vi "Main.vi"() -> ()   [LabVIEW 2012]
uses:
  MeasureDialogButton.ctl
  SourceDialogButton.ctl
  TriggerDialogButton.ctl
  DUTDisplayData.ctl
  DUTDialogButton.ctl
  LogDialogButton.ctl
  driver/Public/Controls/SMU.ctl
  DisplayDataGlobalAction.ctl
  UIActionQueueElement.ctl
  UIAction.ctl
  SetupGlobalAction.ctl
  HardwareActionQueueElement.ctl
  HardwareAction.ctl
  HardwareAbortGlobalAction.ctl
  LogActionQueueElement.ctl
  LogAction.ctl
  DisplayDataChartDialogGlobalAction.ctl
  driver/Keithley-2602.lvlib
  libs/LV-Utilities/LV-Utilities.lvlib
panel:
  in  "CREATE PLOT":bool
  in  "Hardware START":bool
  out "Hardware Running?":bool
  in  "LOG START":bool
  out "Log Running?":bool
  out "Digital IO Port":bool[](array[boolean])
  out "Setup File":path
  in  "RESET":bool
  in  "SAVE":bool
  in  "OPEN":bool
  in  "SHOW LOG DIALOG":T1
  in  "SHOW DUT DIALOG":T2
  in  "SHOW SOURCE DIALOG":T3
  in  "SHOW TRIGGER DIALOG":T4
  in  "SHOW MEASURE DIALOG":T5
  out "System SMU B DUT Display Data":T6[](array[typedef]) {"Resistance (Ohm)" format="%_4p"; "Current (A)" format="%_4p"; "Voltage (V)" format="%_4p"}
  out "System SMU A DUT Display Data":T6[](array[typedef]) {"Resistance (Ohm)" format="%_4p"; "Current (A)" format="%_4p"; "Voltage (V)" format="%_4p"}
  out "Log File":path
  in  "DONE":bool
  # "RUN"
  # "LOG"
  # "DIGITAL IO"
  # "1"
  # "2"
  # "3"
  # "4"
  # "5"
  # "6"
  # "7"
  # "8"
  # "9"
  # "10"
  # "11"
  # "12"
  # "13"
  # "14"
  # "SETUP"
  # "SMU B"
  # "SMU A"
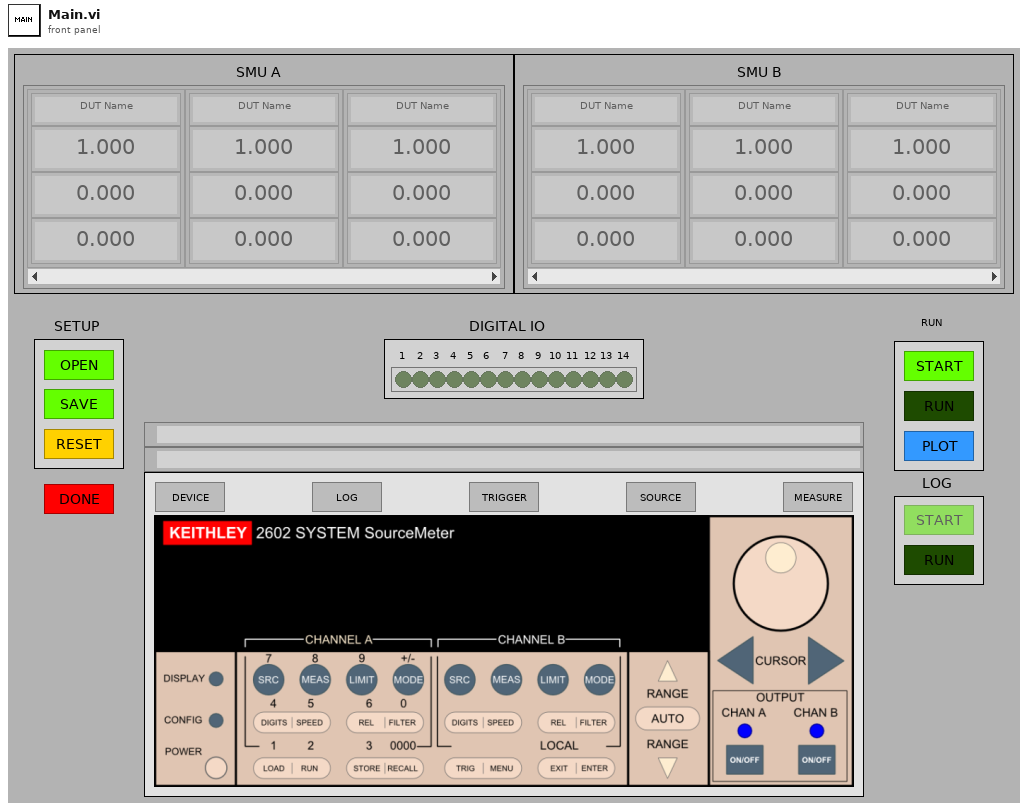
[diagram p1: front panel]
types:
  T1 = typedef "LogDialogButton.ctl" = bool
  T2 = typedef "DUTDialogButton.ctl" = bool
  T3 = typedef "SourceDialogButton.ctl" = bool
  T4 = typedef "TriggerDialogButton.ctl" = bool
  T5 = typedef "MeasureDialogButton.ctl" = bool
  T6 = typedef "DUTDisplayData.ctl" = cluster{"Name":string, "Voltage (V)":dbl, "Current (A)":dbl, "Resistance (Ohm)":dbl}
  T7 = typedef "ExecutableConfiguration.ctl" = cluster{"GPIB ID":u8, "GPIB Board":u8, "Default Data Folder":path, "Default Setup Folder":path}
  T8 = typedef "DataStructures.ctl" = cluster{"Display Data":refnum<notifier>, "Log Data":refnum<queue>}
  T9 = typedef "ActionQueues.ctl" = cluster{"UI Action":refnum<queue>, "Hardware Action":refnum<queue>, "Log Action":refnum<queue>}
  T10 = typedef "DisplayDataGlobalAction.ctl" = enum16{"Get", "Set"}
  T11 = typedef "Keithley-2602.lvlib/SMU.ctl" = enum16{"A", "B"}
  T12 = typedef "SetupGlobalAction.ctl" = enum16{"Get", "Set", "Reset"}
  T13 = enum8{"Enabled", "Disabled", "Disabled and Grayed Out"}
  T14 = typedef "UIActionQueueElement.ctl" = cluster{"Action":T15, "Data":variant}
  T15 = typedef "UIAction.ctl" = enum16{"Initialize", "Configure Trigger", "Configure Measure", "Configure Source", "Configure DUT", "Configure Log", "Configure Open", "Configure Save", "Configure Reset", "Hardware Start", "Hardware Started", "Hardware Stop", "Hardware Stopped", "Log Arm", "Log Start", "Log Started", "Log Stop", "Log Stopped", "Create Chart", "Error", "Shutdown"}
  T16 = typedef "HardwareActionQueueElement.ctl" = cluster{"Action":T17, "Data":variant}
  T17 = typedef "HardwareAction.ctl" = enum16{"Initialize", "Start", "Run", "Stop", "Error", "Shutdown"}
  T18 = typedef "HardwareAbortGlobalAction.ctl" = enum16{"Set", "Get"}
  T19 = typedef "LogActionQueueElement.ctl" = cluster{"Action":T20, "Data":variant}
  T20 = typedef "LogAction.ctl" = enum16{"Initialize", "Start", "Arm", "Create", "Write", "Close", "Rearm", "Stop", "Error", "Shutdown"}
  T21 = typedef "DisplayDataChartDialogGlobalAction.ctl" = enum16{"Create", "Close All"}
  T22 = typedef "HardwareDisplayData.ctl" = cluster{"DUT Names":string[][], "SMU":dbl[][], "Port":bool[]}
  T23 = typedef "Setup.ctl" = cluster{"DUT":T24, "Log":T26, "Trigger":T34, "Sources":T40[], "Measures":T42[]}
  T24 = typedef "DUTConfiguration.ctl" = cluster{"Count":u32, "Wirings":T25[], "Names":string[][]}
  T25 = typedef "Keithley-2602.lvlib/SMUSense.ctl" = enum16{"Local (2-wire)", "Remote (4-wire)", "Calibration"}
  T26 = typedef "LogConfiguration.ctl" = cluster{"Start":T27, "Rollover":T30, "Stop":T32}
  T27 = typedef "LogStartConfiguration.ctl" = cluster{"Trigger Type":T28, "Timer (sec)":dbl, "Digital IO Line":u8, "Digital IO Edge":T29}
  T28 = typedef "LogStartTriggerType.ctl" = enum16{"Immediate", "User", "Timer", "Digital IO"}
  T29 = typedef "LogDigitalIOTriggerEdge.ctl" = enum16{"Rising", "Falling"}
  T30 = typedef "LogRolloverConfiguration.ctl" = cluster{"Trigger Type":T31, "Timer (sec)":dbl, "File Size (MB)":u32, "Digital IO Line":u8, "Digital IO Edge":T29}
  T31 = typedef "LogRolloverTriggerType.ctl" = enum16{"None", "Timer", "File Size", "Digital IO"}
  T32 = typedef "LogStopConfiguration.ctl" = cluster{"Trigger Type":T33, "Timer (sec)":dbl, "File Size (MB)":u32, "Digital IO Line":u8, "Digital IO Edge":T29}
  T33 = typedef "LogStopTriggerType.ctl" = enum16{"None", "User", "Timer", "File Size", "Digital IO"}
  T34 = typedef "TriggerConfiguration.ctl" = cluster{"Input":T35, "Output":T38}
  T35 = typedef "TriggerInputConfiguration.ctl" = cluster{"Type":T36, "Timeout (ms)":u32, "Delay (ms)":u32, "Digital IO Line (1-14)":u8, "Digital IO Mode":T37}
  T36 = typedef "TriggerInputType.ctl" = enum16{"None", "Digital IO", "Bus"}
  T37 = typedef "Keithley-2602.lvlib/TriggerMode.ctl" = enum16{"Falling", "Rising", "Either", "Synchronous"}
  T38 = typedef "TriggerOutputConfiguration.ctl" = cluster{"Type":T39, "Delay (ms)":u32, "Digital IO Line (1-14)":u8, "Digital IO Mode":T37, "Digital IO Pulse Width (sec)":dbl}
  T39 = typedef "TriggerOutputType.ctl" = enum16{"None", "Digital IO", "Bus"}
  T40 = typedef "SourceConfiguration.ctl" = cluster{"Enabled?":bool, "Function":T41, "Level (V or A)":dbl, "Autorange Enabled?":bool, "High Limit (V or A)":dbl, "Low Limit (V or A)":dbl}
  T41 = typedef "SourceFunction.ctl" = enum16{"Voltage", "Current"}
  T42 = typedef "MeasureConfiguration.ctl" = cluster{"Enabled?":bool, "Count":u8, "Interval (sec)":dbl, "Voltage Auto Range Enabled?":bool, "Voltage High Limit (V or A)":dbl, "Voltage Low Limit (V or A)":dbl, "Current Auto Range Enabled?":bool, "Current High Limit (V or A)":dbl, "Current Low Limit (V or A)":dbl}
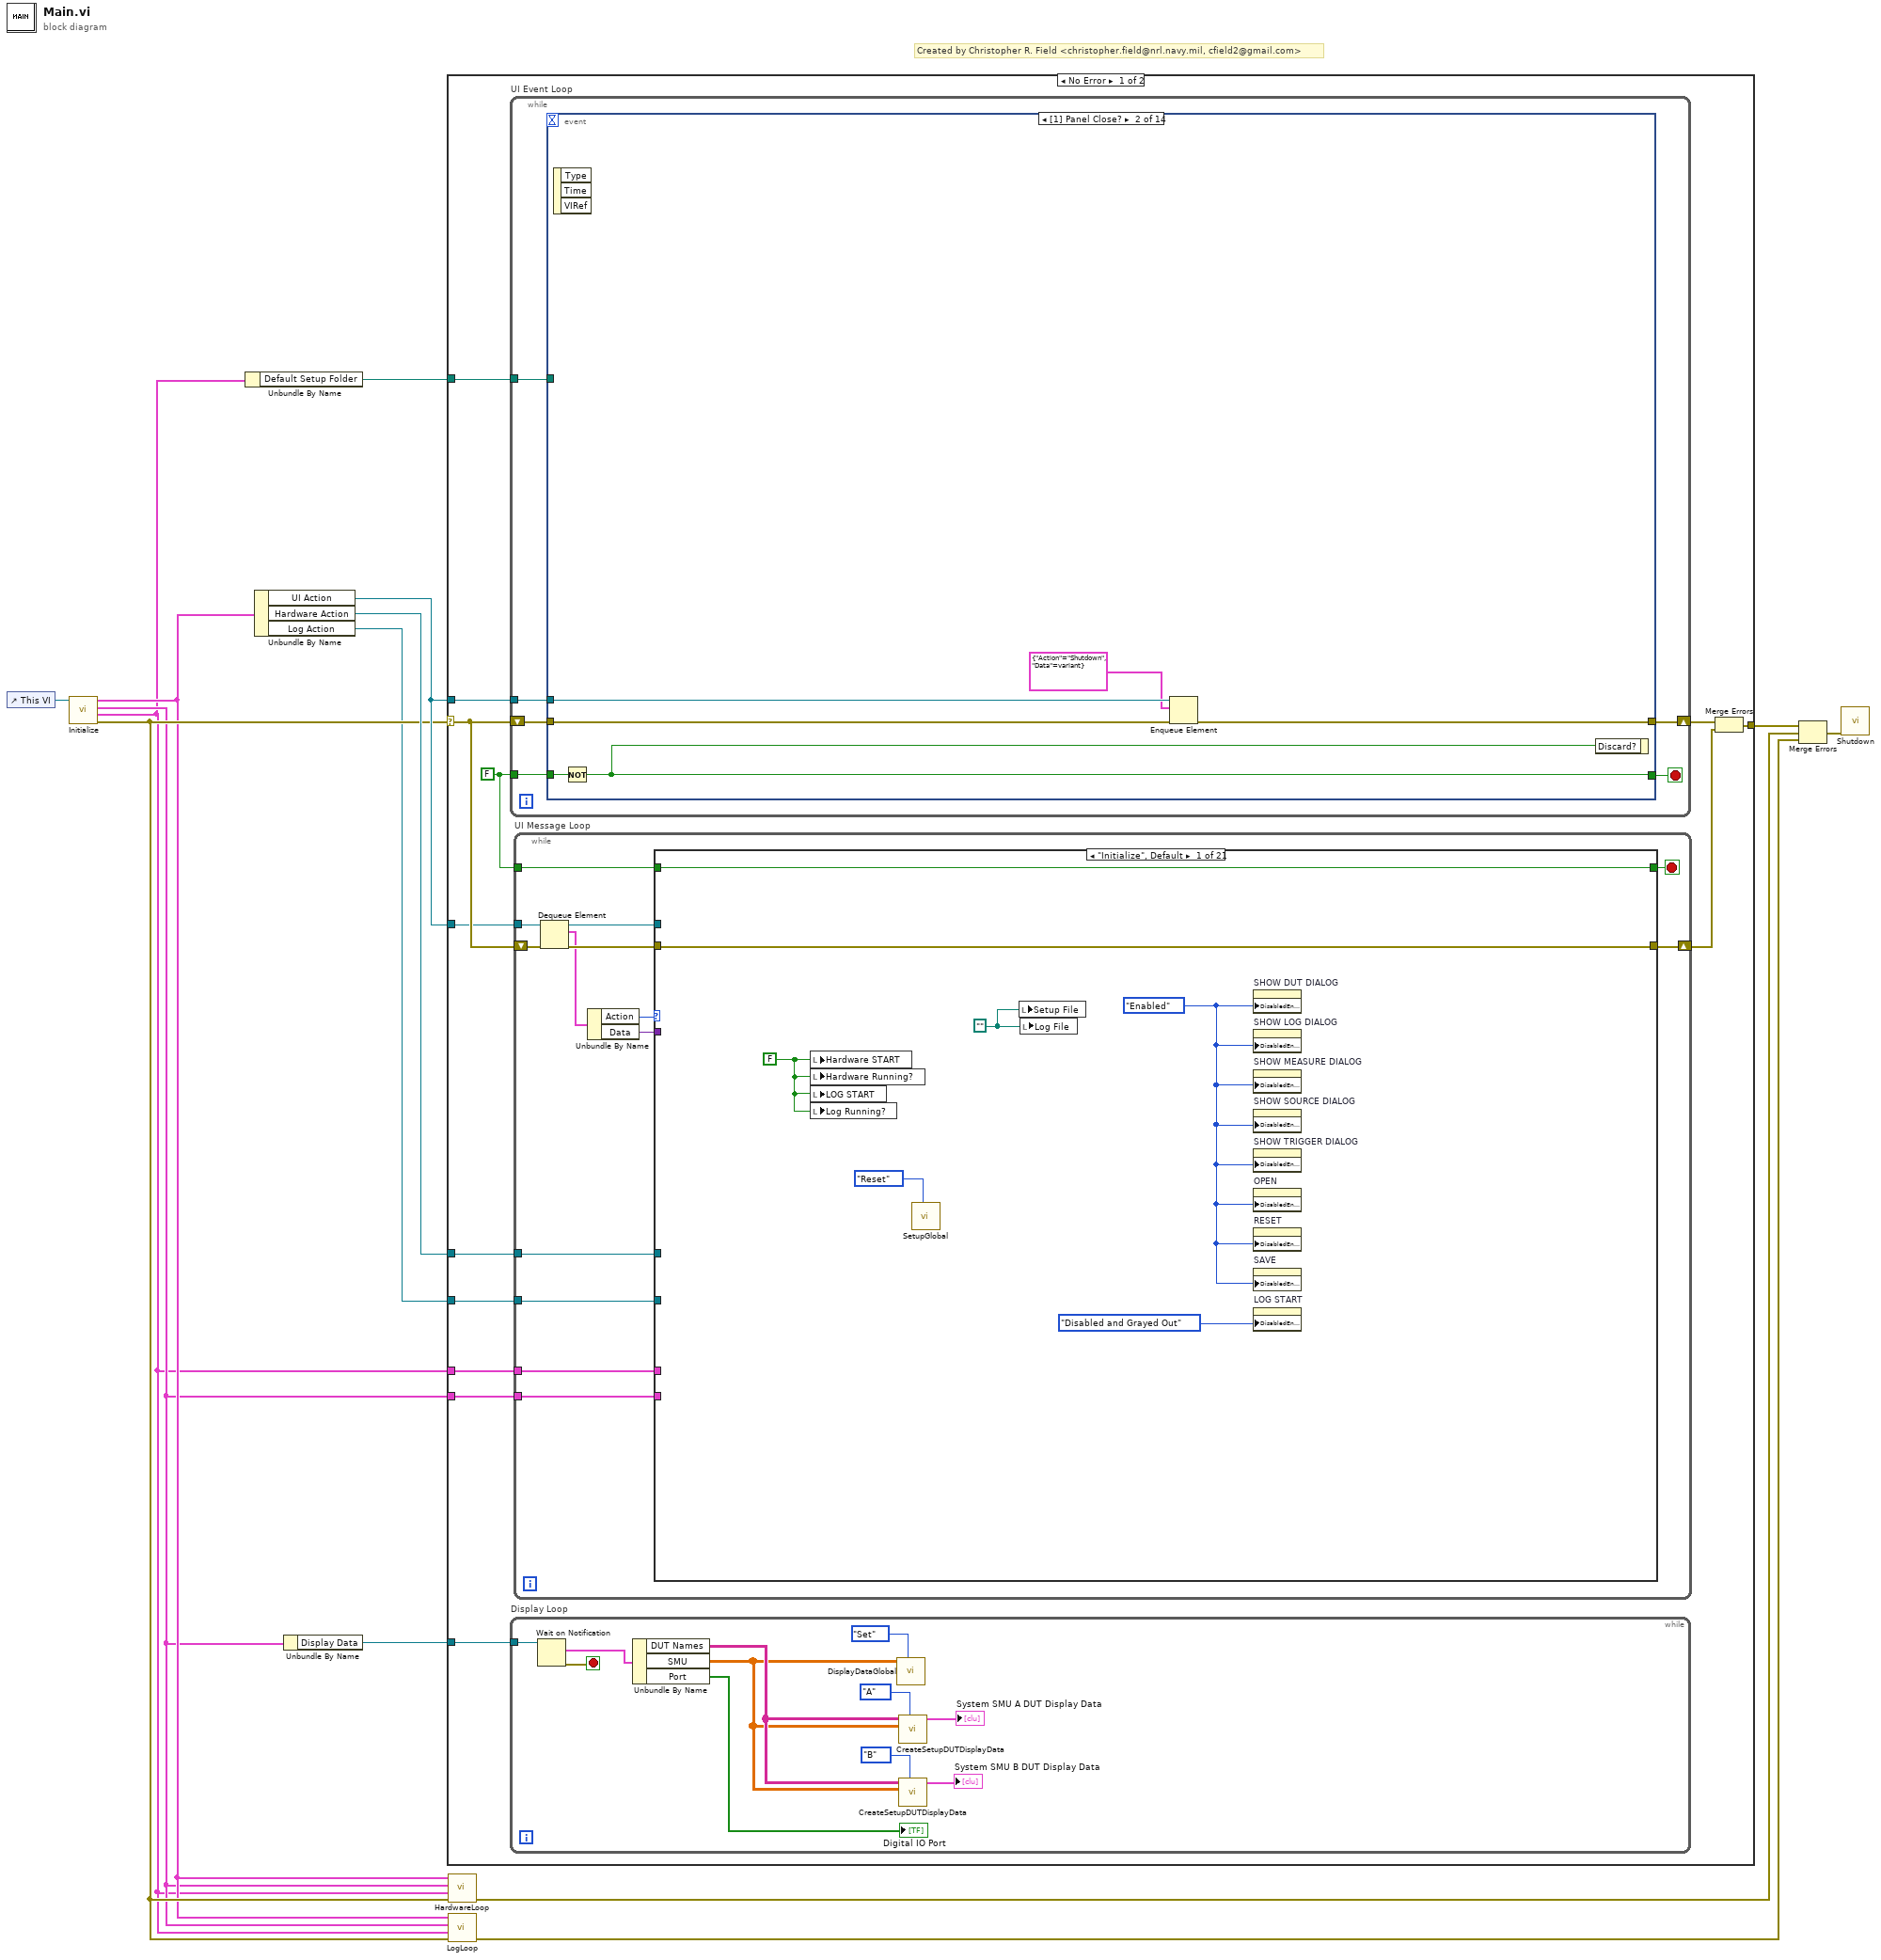
[diagram p0: block diagram]
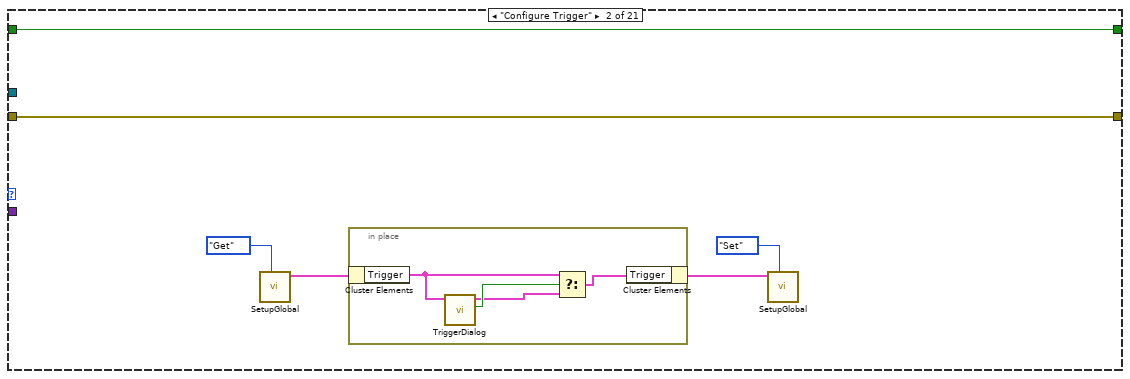
[diagram p2: hidden frame]
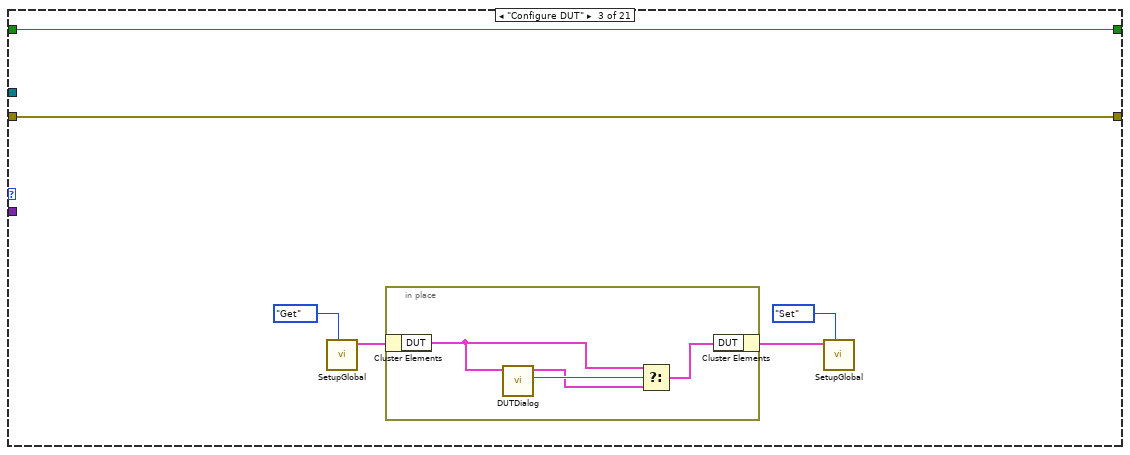
[diagram p3: hidden frame]
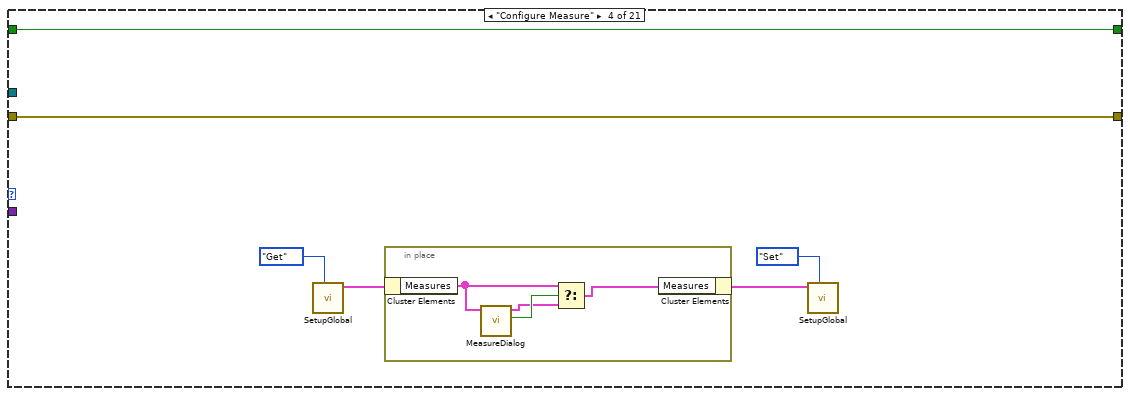
[diagram p4: hidden frame]
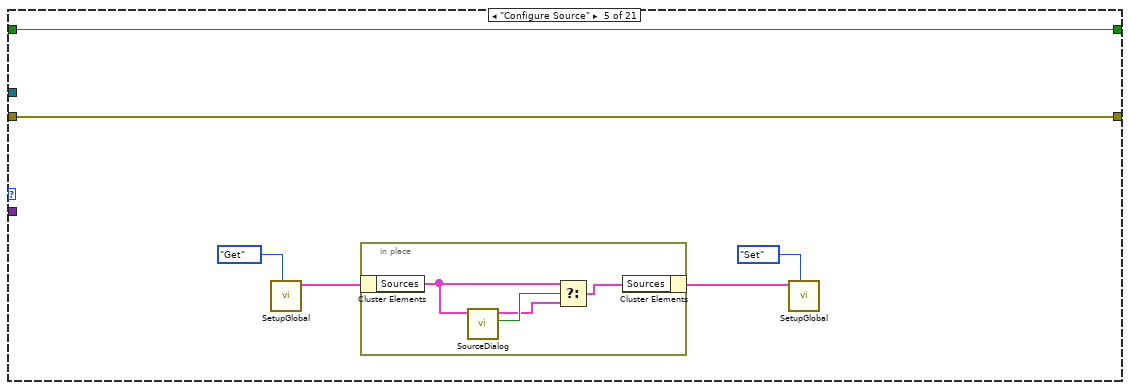
[diagram p5: hidden frame]
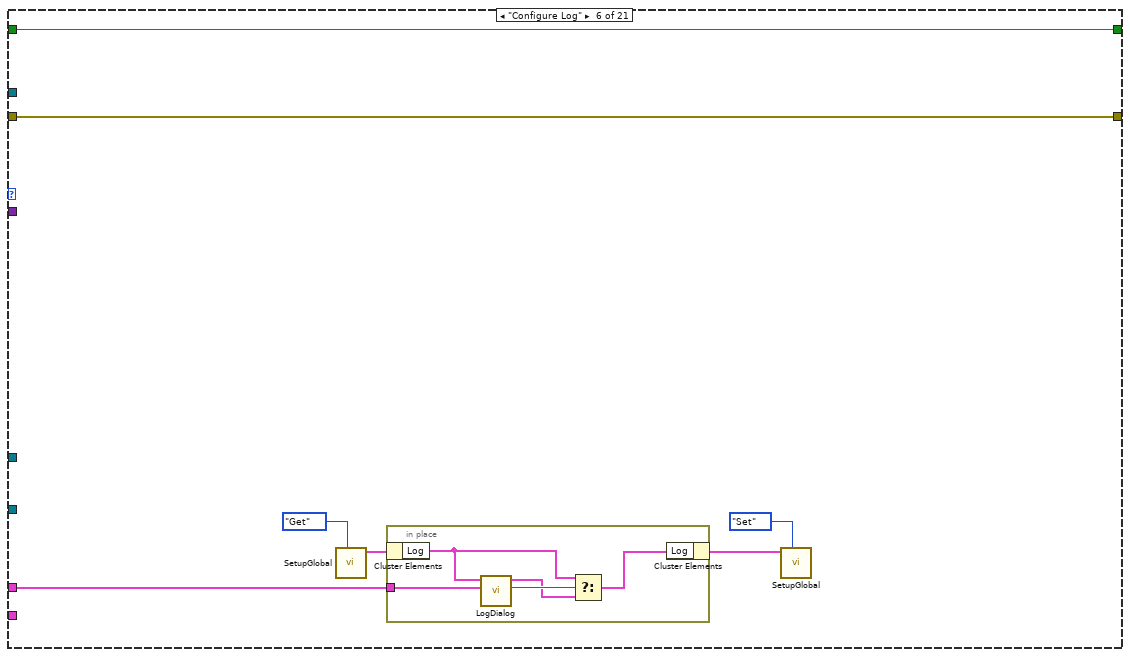
[diagram p6: hidden frame]
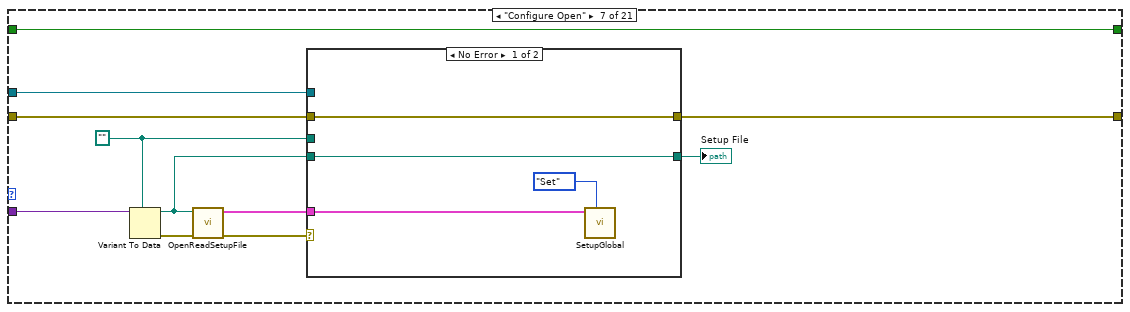
[diagram p7: hidden frame]
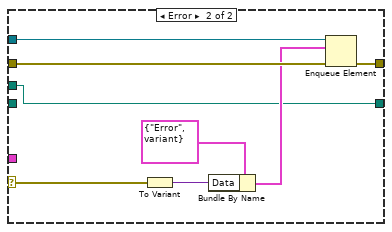
[diagram p8: hidden frame]
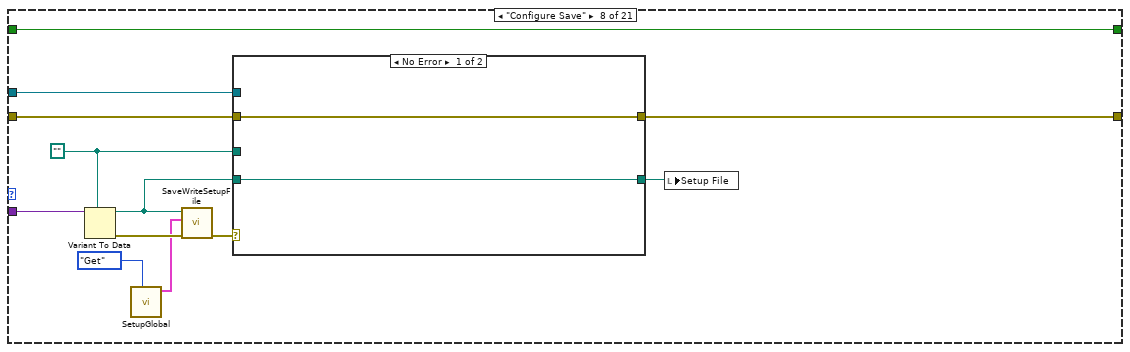
[diagram p9: hidden frame]
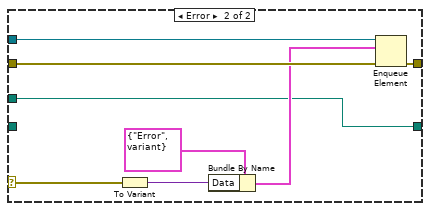
[diagram p10: hidden frame]
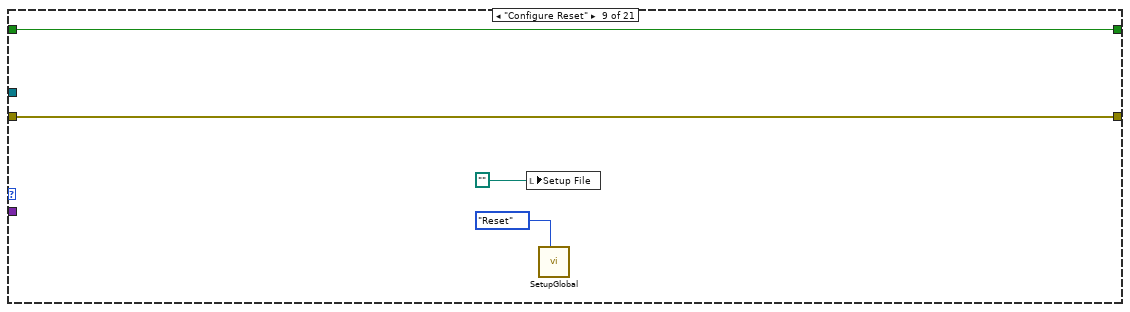
[diagram p11: hidden frame]
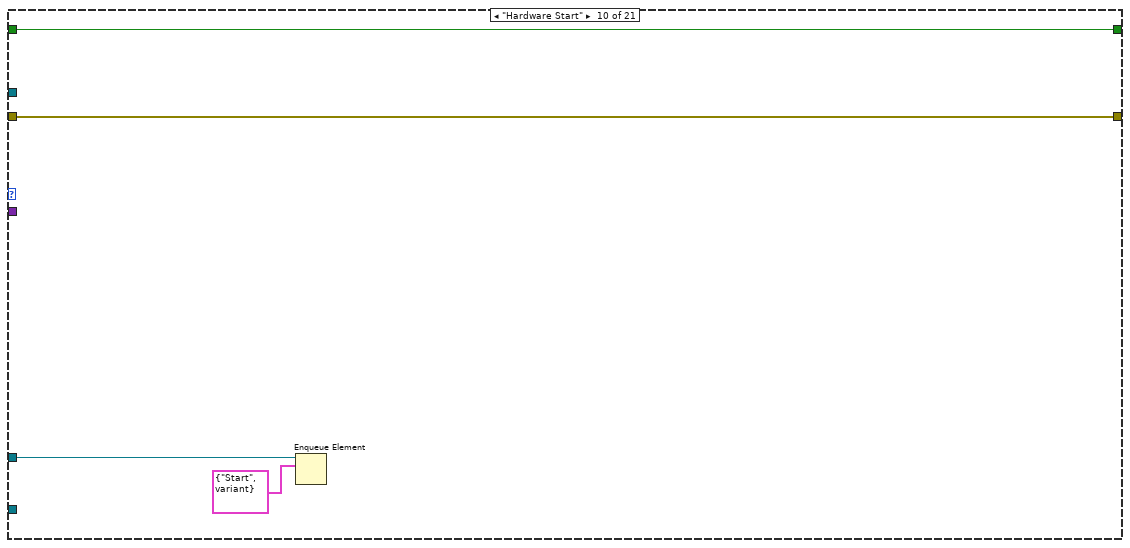
[diagram p12: hidden frame]
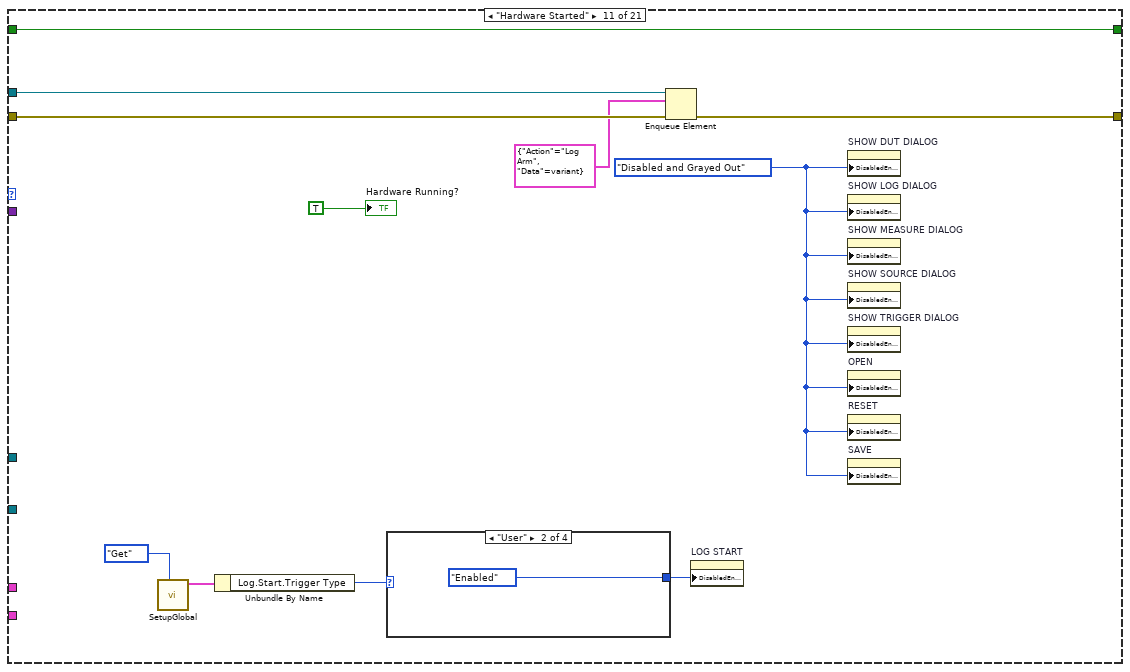
[diagram p13: hidden frame]
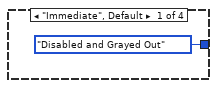
[diagram p14: hidden frame]
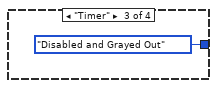
[diagram p15: hidden frame]
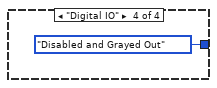
[diagram p16: hidden frame]
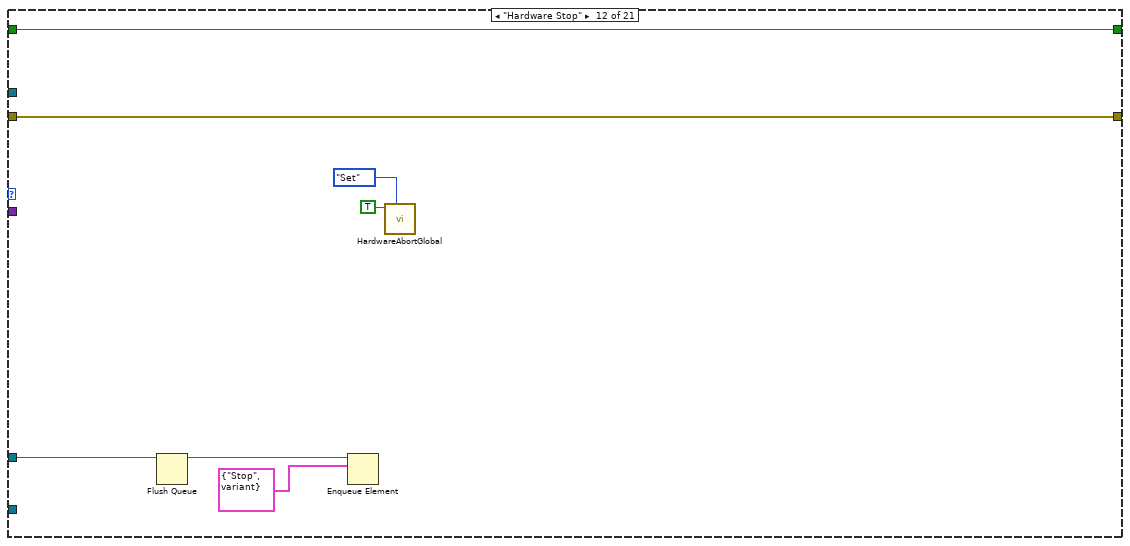
[diagram p17: hidden frame]
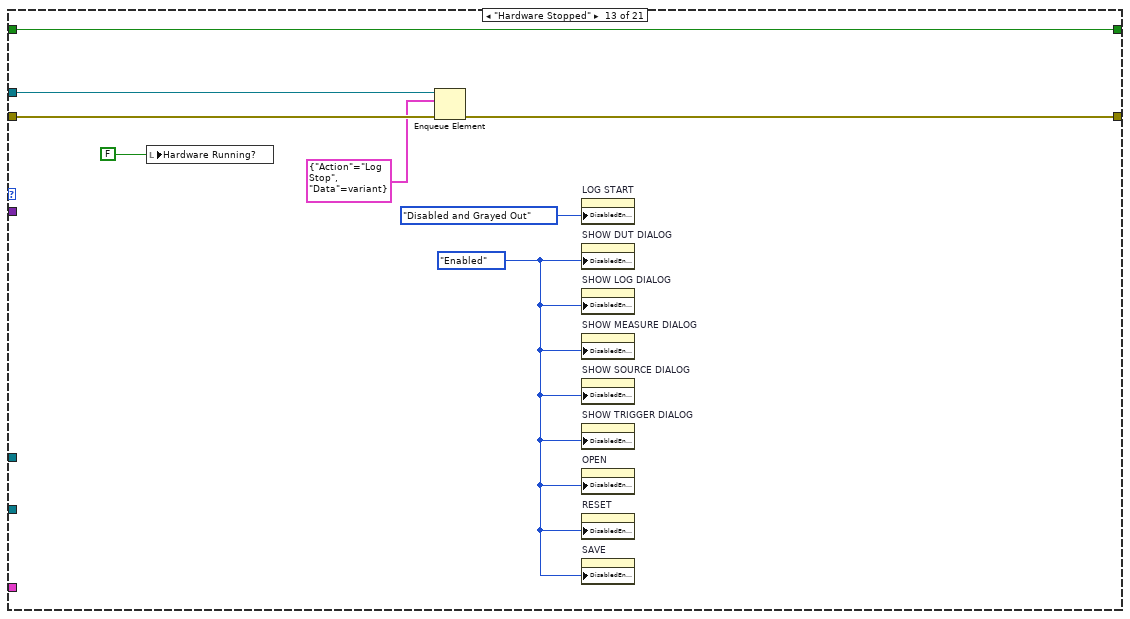
[diagram p18: hidden frame]
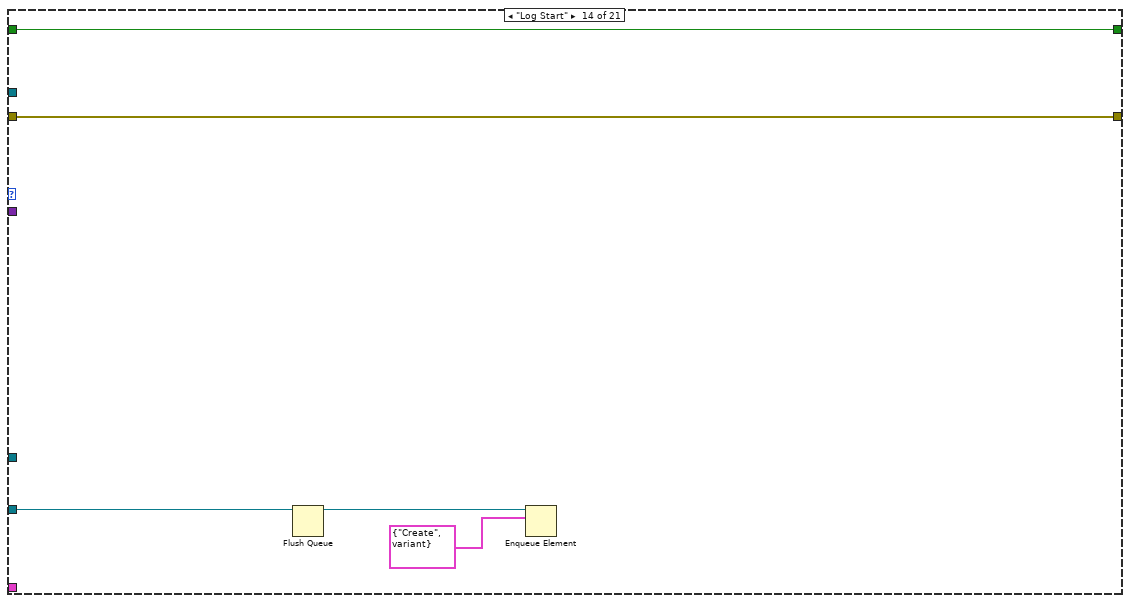
[diagram p19: hidden frame]
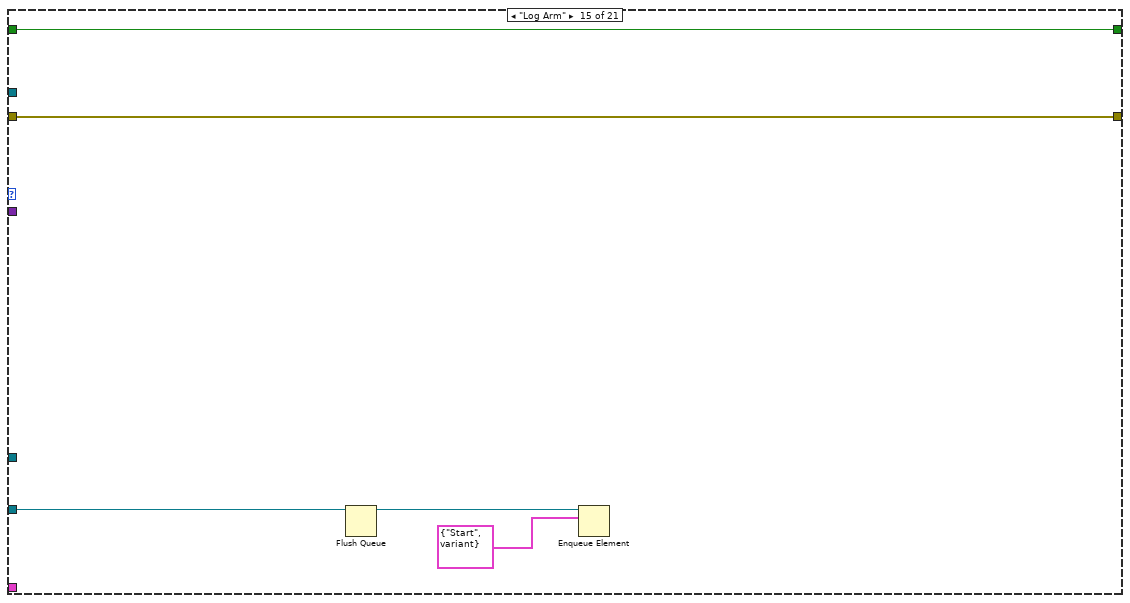
[diagram p20: hidden frame]
diagram:
  # "Created by Christopher R. Field <christopher.field@nrl.navy.mil, cfield2@gmail.com>"
  n1 = control-ref of="This VI"() -> (w1:refnum<vi>)
  n2 = call "Initialize.vi"("VI Ref In"=w1) -> ("Error Out"=w8:errorcluster, "Executable Configuration"=w3:T7, "Data Structures"=w6:T8, "Action Queues"=w7:T9)  [unwired: 7 in]
  n3 = Unbundle By Name(w3) -> ("Default Setup Folder"=w2:path)
  n4 = Unbundle By Name(w7) -> ("UI Action"=w14:refnum<queue>, "Hardware Action"=w10:refnum<queue>, "Log Action"=w4:refnum<queue>)
  n5 = Unbundle By Name(w6) -> ("Display Data"=w9:refnum<notifier>)
  n6 = case shown="No Error" w8 {
    selector: w8 -> [w25 w378]
    tunnel: [w26 w378] -> w13
    tunnel: w14 -> [w22 _]
    tunnel: w14 -> [w21 _]
    tunnel: w10 -> [w20 _]
    tunnel: w9 -> [w19 _]
    tunnel: w6 -> [w18 _]
    tunnel: w3 -> [w17 _]
    tunnel: w4 -> [w16 _]
    tunnel: w2 -> [w15 _]
    frame No Error {
      w23 = FALSE
      n7 = while "UI Event Loop" {
        tunnel: w23 -> [w272]
        shift-right: [w269] -> w27
        shift-left: w25 -> [w270]
        tunnel: w21 -> [w268]
        tunnel: w15 -> [w267]
        stop <- w271 stop-if-true
        n8 = event shown="[1] Panel Close?" {
          selector: _ -> [_ _ _ _ _ _ _ _ _ _ _ _ _ _]
          dyn-events: _ -> [_ _ _ _ _ _ _ _ _ _ _ _ _ _]
          timeout: _ -> [_ _ _ _ _ _ _ _ _ _ _ _ _ _]
          tunnel: w272 -> [w274 w280 w285 w299 w315 w331 w336 w341 w343 w357 w362 w364 w372 w374]
          tunnel: [w274 w279 w285 w299 w315 w331 w336 w341 w343 w356 w362 w364 w372 w374] -> w271
          tunnel: w270 -> [w273 w276 w287 w290 w317 w329 w334 w339 w345 w352 w360 w366 w370 w376]
          tunnel: [w273 w277 w286 w291 w316 w328 w333 w338 w344 w355 w359 w365 w369 w375] -> w269
          tunnel: w268 -> [_ w278 w288 w292 w318 w330 w335 w340 w346 w353 w361 w367 w371 w377]
          tunnel: w267 -> [_ _ _ w289 w308 _ _ _ _ _ _ _ _ _]
          event Timeout {
            n9 = event-data() -> ()  [unwired: 1 in, 2 out]
          }
          event Panel Close? {
            n10 = event-data() -> ()  [unwired: 1 in, 3 out]
            n11 = Not(x=w280) -> (.not. x?=w279:bool)
            n12 = Enqueue Element(queue=w278, element=T14 {"Action"=enum."Shutdown", "Data"=variant}, error in (no error)=w276) -> (error out=w277:errorcluster)  [unwired: 1 in, 2 out]
            n13 = event-data("Discard?"=w279) -> ()  [unwired: 1 in, 1 out]
          }
          event "LOG START": Value Change {
            n14 = event-data() -> ()  [unwired: 1 in, 5 out]
            n15 = Select(t=T14 {"Action"=enum."Log Start", "Data"=variant} ("element"), s="LOG START", f=T14 {"Action"=enum."Log Stop", "Data"=variant} ("element")) -> (s? t:f=w281:T14)
            n16 = Enqueue Element(queue=w288, element=w281, error in (no error)=w287) -> (error out=w286:errorcluster)  [unwired: 1 in, 2 out]
          }
          event "OPEN": Value Change {
            n17 = event-data() -> ()  [unwired: 1 in, 5 out]
            n18 = call "SelectFile.vi"("Button Label"="Open", "Prompt"="Select Setup File", "File Description"="Setup File", "File Extension (.*)"=".xml", "Start Path"=w289) -> ("Cancelled?"=w294:bool, "Selected File Path"=w293:path)  [unwired: 4 in, 1 out]
            n19 = case shown="False" w294 {
              tunnel: w292 -> [w306 _]
              tunnel: w290 -> [w305 w307]
              tunnel: [w304 w307] -> w291
              tunnel: w293 -> [w301 _]
              frame False {
                n20 = To Variant(anything=w301) -> (Variant=w302:variant)
                n21 = Bundle By Name(cluster=T14 {"Action"=enum."Configure Open", "Data"=variant} ("element"), "Data"=w302) -> (w300:T14)
                n22 = Enqueue Element(queue=w306, element=w300, error in (no error)=w305) -> (error out=w304:errorcluster)  [unwired: 1 in, 2 out]
              }
              frame True {
              }
            }
          }
          event "SAVE": Value Change {
            n23 = event-data() -> ()  [unwired: 1 in, 5 out]
            n24 = call "SelectFile.vi"("Button Label"="Save", "Prompt"="Select Setup File", "File Description"="Setup File", "File Extension (.*)"=".xml", "Start Path"=w308) -> ("Cancelled?"=w310:bool, "Selected File Path"=w309:path)  [unwired: 4 in, 1 out]
            n25 = case shown="False" w310 {
              tunnel: w318 -> [w325 _]
              tunnel: w317 -> [w324 w326]
              tunnel: [w323 w326] -> w316
              tunnel: w309 -> [w320 _]
              frame False {
                n26 = To Variant(anything=w320) -> (Variant=w321:variant)
                n27 = Bundle By Name(cluster=T14 {"Action"=enum."Configure Save", "Data"=variant} ("element"), "Data"=w321) -> (w319:T14)
                n28 = Enqueue Element(queue=w325, element=w319, error in (no error)=w324) -> (error out=w323:errorcluster)  [unwired: 1 in, 2 out]
              }
              frame True {
              }
            }
          }
          event "RESET": Value Change {
            n29 = event-data() -> ()  [unwired: 1 in, 5 out]
            n30 = Enqueue Element(queue=w330, element=T14 {"Action"=enum."Configure Reset", "Data"=variant}, error in (no error)=w329) -> (error out=w328:errorcluster)  [unwired: 1 in, 2 out]
          }
          event Value Change {
            n31 = event-data() -> ()  [unwired: 1 in, 1 out]
            n32 = Enqueue Element(queue=w335, element=T14 {"Action"=enum."Configure Measure", "Data"=variant}, error in (no error)=w334) -> (error out=w333:errorcluster)  [unwired: 1 in, 2 out]
          }
          event Value Change {
            n33 = event-data() -> ()  [unwired: 1 in, 5 out]
            n34 = Enqueue Element(queue=w340, element=T14 {"Action"=enum."Configure Source", "Data"=variant}, error in (no error)=w339) -> (error out=w338:errorcluster)  [unwired: 1 in, 2 out]
          }
          event "Hardware START": Value Change {
            n35 = event-data() -> ()  [unwired: 1 in, 1 out]
            n36 = Select(t=T14 {"Action"=enum."Hardware Start", "Data"=variant} ("UI Action Queue Element"), s="Hardware START", f=T14 {"Action"=enum."Hardware Stop", "Data"=variant} ("UI Action Queue Element")) -> (s? t:f=w342:T14)
            n37 = Enqueue Element(queue=w346, element=w342, error in (no error)=w345) -> (error out=w344:errorcluster)  [unwired: 1 in, 2 out]
          }
          event "DONE": Value Change {
            n38 = event-data() -> ()  [unwired: 1 in, 5 out]
            n39 = Not(x=w357) -> (.not. x?=w356:bool)
            n40 = Flush Queue(queue=w353, error in (no error)=w352) -> (queue out=w350:refnum<queue>, error out=w351:errorcluster)  [unwired: 1 out]
            n41 = Enqueue Element(queue=w350, element=T14 {"Action"=enum."Shutdown", "Data"=variant}, error in (no error)=w351) -> (error out=w355:errorcluster)  [unwired: 1 in, 2 out]
          }
          event Value Change {
            n42 = event-data() -> ()  [unwired: 1 in, 5 out]
            n43 = Enqueue Element(queue=w361, element=T14 {"Action"=enum."Configure Trigger", "Data"=variant}, error in (no error)=w360) -> (error out=w359:errorcluster)  [unwired: 1 in, 2 out]
          }
          event "CREATE PLOT": Value Change {
            n44 = event-data() -> ()  [unwired: 1 in, 5 out]
            n45 = Enqueue Element(queue=w367, element=T14 {"Action"=enum."Create Chart", "Data"=variant} ("UI Action Queue Element"), error in (no error)=w366) -> (error out=w365:errorcluster)  [unwired: 1 in, 2 out]
          }
          event Value Change {
            n46 = event-data() -> ()  [unwired: 1 in, 5 out]
            n47 = Enqueue Element(queue=w371, element=T14 {"Action"=enum."Configure DUT", "Data"=variant}, error in (no error)=w370) -> (error out=w369:errorcluster)  [unwired: 1 in, 2 out]
          }
          event Value Change {
            n48 = event-data() -> ()  [unwired: 1 in, 5 out]
            n49 = Enqueue Element(queue=w377, element=T14 {"Action"=enum."Configure Log", "Data"=variant}, error in (no error)=w376) -> (error out=w375:errorcluster)  [unwired: 1 in, 2 out]
          }
        }
      }
      n50 = while "Display Loop" {
        tunnel: w19 -> [w38]
        stop <- w37 stop-if-true
        n51 = Wait on Notification(notifier=w38) -> (notification=w36:T22, error out=w37:errorcluster)  [unwired: 3 in, 2 out]
        n52 = Unbundle By Name(w36) -> ("DUT Names"=w32:string[][], "SMU"=w29:dbl[][], "Port"=→"Digital IO Port":bool[])
        n53 = call "DisplayDataGlobal.vi"("Action"=DisplayDataGlobalAction."Set", "Set Value"=w29) -> ()  [unwired: 9 in, 1 out]
        n54 = call "CreateSetupDUTDisplayData.vi"("SMU"=SMU."A", "SMU Data"=w29, "DUT Names"=w32) -> ("DUT Display Data"=→"System SMU A DUT Display Data":T6[])  [unwired: 8 in]
        n55 = call "CreateSetupDUTDisplayData.vi"("SMU"=SMU."B", "SMU Data"=w29, "DUT Names"=w32) -> ("DUT Display Data"=→"System SMU B DUT Display Data":T6[])  [unwired: 8 in]
      }
      n56 = while "UI Message Loop" {
        shift-right: [w51] -> w24
        shift-left: w25 -> [w49]
        tunnel: w23 -> [w52]
        tunnel: w22 -> [w48]
        tunnel: w20 -> [w42]
        tunnel: w18 -> [w41]
        tunnel: w17 -> [w40]
        tunnel: w16 -> [w39]
        stop <- w50 stop-if-true
        n57 = Dequeue Element(queue=w48, error in (no error)=w49) -> (queue out=w46:refnum<queue>, element=w45:T14, error out=w47:errorcluster)  [unwired: 1 in, 1 out]
        n58 = Unbundle By Name(w45) -> ("Action"=w44:T15, "Data"=w43:variant)
        n59 = case shown="\"Initialize\", Default" w44 {
          tunnel: w52 -> [w59 w65 w75 w85 w95 w106 w122 w146 w160 w164 w175 w186 w194 w199 w204 w214 w225 w232 w243 w247 w262]
          tunnel: w47 -> [w58 w64 w74 w84 w94 w105 w115 w140 w159 w163 w171 w185 w191 w198 w201 w213 w224 w233 w242 w245 w259]
          tunnel: [w58 w64 w74 w84 w94 w105 w114 w139 w159 w163 w170 w185 w190 w198 w201 w213 w224 w233 w242 w245 w258] -> w51
          tunnel: [w59 w65 w75 w85 w95 w106 w122 w146 w160 w164 w175 w186 w194 w199 w204 w214 w225 w232 w243 w247 w261] -> w50
          tunnel: w46 -> [_ _ _ _ _ _ w116 w141 _ _ w172 _ w192 _ _ _ _ _ _ _ w260]
          tunnel: w43 -> [_ _ _ _ _ _ w121 w145 _ _ _ _ _ _ _ w212 _ _ _ w246 _]
          tunnel: w42 -> [_ _ _ _ _ _ _ _ _ w162 _ w183 _ _ _ _ _ _ _ _ w257]
          tunnel: w41 -> [_ _ _ _ _ _ _ _ _ _ _ _ _ _ _ _ _ _ _ _ _]
          tunnel: w40 -> [_ _ _ _ _ w104 _ _ _ _ _ _ _ _ _ _ _ _ _ _ _]
          tunnel: w39 -> [_ _ _ _ _ _ _ _ _ _ _ _ _ w197 w202 _ w223 _ _ _ w255]
          frame "Initialize", Default {
            w54 = T13."Enabled" ("Disabled")
            w55 = path ""
            w57 = FALSE ("START")
            n60 = local write "Hardware START"(w57) -> ()
            n61 = local write "Hardware Running?"(w57) -> ()
            n62 = local write "LOG START"(w57) -> ()
            n63 = local write "Log Running?"(w57) -> ()
            n64 = call "SetupGlobal.vi"("Action"=SetupGlobalAction."Reset") -> ()  [unwired: 10 in, 1 out]
            n65 = local write "Setup File"(w55) -> ()
            n66 = local write "Log File"(w55) -> ()
            n67 = property on="SHOW DUT DIALOG" class="Bool"("DisabledEnum"=w54) -> ()  [unwired: 2 in, 2 out]
            n68 = property on="SHOW LOG DIALOG" class="Bool"("DisabledEnum"=w54) -> ()  [unwired: 2 in, 2 out]
            n69 = property on="SHOW MEASURE DIALOG" class="Bool"("DisabledEnum"=w54) -> ()  [unwired: 2 in, 2 out]
            n70 = property on="SHOW SOURCE DIALOG" class="Bool"("DisabledEnum"=w54) -> ()  [unwired: 2 in, 2 out]
            n71 = property on="SHOW TRIGGER DIALOG" class="Bool"("DisabledEnum"=w54) -> ()  [unwired: 2 in, 2 out]
            n72 = property on="OPEN" class="Bool"("DisabledEnum"=w54) -> ()  [unwired: 2 in, 2 out]
            n73 = property on="RESET" class="Bool"("DisabledEnum"=w54) -> ()  [unwired: 2 in, 2 out]
            n74 = property on="SAVE" class="Bool"("DisabledEnum"=w54) -> ()  [unwired: 2 in, 2 out]
            n75 = property on="LOG START" class="Bool (strict)"("DisabledEnum"=T13."Disabled and Grayed Out" ("Disabled")) -> ()  [unwired: 2 in, 2 out]
          }
          frame "Configure Trigger" {
            n76 = call "SetupGlobal.vi"("Action"=SetupGlobalAction."Get") -> ("Value Out"=w62:T23)  [unwired: 10 in]
            n77 = in-place {
              n78 = in-place-cluster #1(w62) -> ("Trigger"=w66:T34)
              n79 = call "TriggerDialog.vi"("Trigger Configuration In"=w66) -> ("Cancelled"=w69:bool, "Trigger Configuration Out"=w68:T34)  [unwired: 8 in, 1 out]
              n80 = Select(t=w66, s=w69, f=w68) -> (s? t:f=w67:T34)
              n81 = in-place-cluster #1("Trigger"=w67) -> (w61:T23)
            }
            n82 = call "SetupGlobal.vi"("Action"=SetupGlobalAction."Set", "Set Value"=w61) -> ()  [unwired: 9 in, 1 out]
          }
          frame "Configure DUT" {
            n83 = call "SetupGlobal.vi"("Action"=SetupGlobalAction."Get") -> ("Value Out"=w72:T23)  [unwired: 10 in]
            n84 = in-place {
              n85 = in-place-cluster #2(w72) -> ("DUT"=w76:T24)
              n86 = call "DUTDialog.vi"("DUT Configuration In"=w76) -> ("Cancelled?"=w79:bool, "DUT Configuration Out"=w78:T24)  [unwired: 8 in, 1 out]
              n87 = Select(t=w76, s=w79, f=w78) -> (s? t:f=w77:T24)
              n88 = in-place-cluster #2("DUT"=w77) -> (w70:T23)
            }
            n89 = call "SetupGlobal.vi"("Action"=SetupGlobalAction."Set", "Set Value"=w70) -> ()  [unwired: 9 in, 1 out]
          }
          frame "Configure Measure" {
            n90 = call "SetupGlobal.vi"("Action"=SetupGlobalAction."Get") -> ("Value Out"=w82:T23)  [unwired: 10 in]
            n91 = in-place {
              n92 = in-place-cluster #3(w82) -> ("Measures"=w86:T42[])
              n93 = call "MeasureDialog.vi"("Measure Configuration In"=w86) -> ("Cancelled?"=w89:bool, "Measure Configuration Out"=w87:T42[])  [unwired: 8 in, 1 out]
              n94 = Select(t=w86, s=w89, f=w87) -> (s? t:f=w88:T42[])
              n95 = in-place-cluster #3("Measures"=w88) -> (w80:T23)
            }
            n96 = call "SetupGlobal.vi"("Action"=SetupGlobalAction."Set", "Set Value"=w80) -> ()  [unwired: 9 in, 1 out]
          }
          frame "Configure Source" {
            n97 = call "SetupGlobal.vi"("Action"=SetupGlobalAction."Get") -> ("Value Out"=w92:T23)  [unwired: 10 in]
            n98 = in-place {
              n99 = in-place-cluster #4(w92) -> ("Sources"=w96:T40[])
              n100 = call "SourceDialog.vi"("Source Configurations In"=w96) -> ("Cancelled?"=w99:bool, "Source Configurations Out"=w98:T40[])  [unwired: 8 in, 1 out]
              n101 = Select(t=w96, s=w99, f=w98) -> (s? t:f=w97:T40[])
              n102 = in-place-cluster #4("Sources"=w97) -> (w90:T23)
            }
            n103 = call "SetupGlobal.vi"("Action"=SetupGlobalAction."Set", "Set Value"=w90) -> ()  [unwired: 9 in, 1 out]
          }
          frame "Configure Log" {
            n104 = call "SetupGlobal.vi"("Action"=SetupGlobalAction."Get") -> ("Value Out"=w102:T23)  [unwired: 10 in]
            n105 = in-place {
              in-place-border: w104 -> [w108]
              n106 = in-place-cluster #5(w102) -> ("Log"=w107:T26)
              n107 = call "LogDialog.vi"("Executable Configuration"=w108, "Log Configuration In"=w107) -> ("Cancelled?"=w111:bool, "Log Configuration Out"=w110:T26)  [unwired: 7 in, 1 out]
              n108 = Select(t=w107, s=w111, f=w110) -> (s? t:f=w109:T26)
              n109 = in-place-cluster #5("Log"=w109) -> (w100:T23)
            }
            n110 = call "SetupGlobal.vi"("Action"=SetupGlobalAction."Set", "Set Value"=w100) -> ()  [unwired: 9 in, 1 out]
          }
          frame "Configure Open" {
            w112 = path ""
            n111 = Variant To Data(type=w112, Variant=w121) -> (data=w117:path, error out=w120:errorcluster)  [unwired: 1 in]
            n112 = call "OpenReadSetupFile.vi"("Error In"=w120, "Setup File"=w117) -> ("Error Out"=w119:errorcluster, "Setup"=w118:T23)  [unwired: 8 in]
            n113 = case shown="No Error" w119 {
              selector: w119 -> [_ w129]
              tunnel: w118 -> [w124 _]
              tunnel: w117 -> [w123 _]
              tunnel: w116 -> [_ w134]
              tunnel: w115 -> [w126 w133]
              tunnel: [w126 w132] -> w114
              tunnel: [w123 w127] -> w113
              tunnel: w112 -> [_ w127]
              frame No Error {
                n114 = call "SetupGlobal.vi"("Action"=SetupGlobalAction."Set", "Set Value"=w124) -> ()  [unwired: 9 in, 1 out]
              }
              frame Error {
                n115 = To Variant(anything=w129) -> (Variant=w130:variant)
                n116 = Bundle By Name(cluster=T14 {"Action"=enum."Error", "Data"=variant} ("element"), "Data"=w130) -> (w128:T14)
                n117 = Enqueue Element(queue=w134, element=w128, error in (no error)=w133) -> (error out=w132:errorcluster)  [unwired: 1 in, 2 out]
              }
            }
            "Setup File" <- w113
          }
          frame "Configure Save" {
            w135 = path ""
            n118 = Variant To Data(type=w135, Variant=w145) -> (data=w143:path, error out=w144:errorcluster)  [unwired: 1 in]
            n119 = call "SetupGlobal.vi"("Action"=SetupGlobalAction."Get") -> ("Value Out"=w137:T23)  [unwired: 10 in]
            n120 = call "SaveWriteSetupFile.vi"("Error In"=w144, "Setup"=w137, "Save File"=w143) -> ("Error Out"=w142:errorcluster)  [unwired: 8 in]
            n121 = case shown="No Error" w142 {
              selector: w142 -> [_ w151]
              tunnel: w143 -> [w147 _]
              tunnel: w141 -> [_ w156]
              tunnel: w140 -> [w148 w155]
              tunnel: [w148 w154] -> w139
              tunnel: [w147 w149] -> w136
              tunnel: w135 -> [_ w149]
              frame No Error {
              }
              frame Error {
                n122 = To Variant(anything=w151) -> (Variant=w152:variant)
                n123 = Bundle By Name(cluster=T14 {"Action"=enum."Error", "Data"=variant} ("element"), "Data"=w152) -> (w150:T14)
                n124 = Enqueue Element(queue=w156, element=w150, error in (no error)=w155) -> (error out=w154:errorcluster)  [unwired: 1 in, 2 out]
              }
            }
            n125 = local write "Setup File"(w136) -> ()
          }
          frame "Configure Reset" {
            n126 = local write "Setup File"(path "") -> ()
            n127 = call "SetupGlobal.vi"("Action"=SetupGlobalAction."Reset") -> ()  [unwired: 10 in, 1 out]
          }
          frame "Hardware Start" {
            n128 = Enqueue Element(queue=w162, element=T16 {"Action"=enum."Start", "Data"=variant} ("Hardware Action Queue Element")) -> ()  [unwired: 2 in, 3 out]
          }
          frame "Hardware Started" {
            w168 = T13."Disabled and Grayed Out" ("Disabled")
            n129 = call "SetupGlobal.vi"("Action"=SetupGlobalAction."Get") -> ("Value Out"=w166:T23)  [unwired: 10 in]
            n130 = Unbundle By Name(w166) -> ("Log.Start.Trigger Type"=w165:T28)
            n131 = case shown="\"User\"" w165 {
              tunnel: [T13."Disabled and Grayed Out" ("Disabled") T13."Enabled" ("Disabled") T13."Disabled and Grayed Out" ("Disabled") T13."Disabled and Grayed Out" ("Disabled")] -> w173
              frame "Immediate", Default {
              }
              frame "User" {
              }
              frame "Timer" {
              }
              frame "Digital IO" {
              }
            }
            n132 = Enqueue Element(queue=w172, element=T14 {"Action"=enum."Log Arm", "Data"=variant}, error in (no error)=w171) -> (error out=w170:errorcluster)  [unwired: 1 in, 2 out]
            n133 = property on="LOG START" class="Bool (strict)"("DisabledEnum"=w173) -> ()  [unwired: 2 in, 2 out]
            n134 = property on="SHOW DUT DIALOG" class="Bool"("DisabledEnum"=w168) -> ()  [unwired: 2 in, 2 out]
            n135 = property on="SHOW LOG DIALOG" class="Bool"("DisabledEnum"=w168) -> ()  [unwired: 2 in, 2 out]
            n136 = property on="SHOW MEASURE DIALOG" class="Bool"("DisabledEnum"=w168) -> ()  [unwired: 2 in, 2 out]
            n137 = property on="SHOW SOURCE DIALOG" class="Bool"("DisabledEnum"=w168) -> ()  [unwired: 2 in, 2 out]
            n138 = property on="SHOW TRIGGER DIALOG" class="Bool"("DisabledEnum"=w168) -> ()  [unwired: 2 in, 2 out]
            n139 = property on="OPEN" class="Bool"("DisabledEnum"=w168) -> ()  [unwired: 2 in, 2 out]
            n140 = property on="RESET" class="Bool"("DisabledEnum"=w168) -> ()  [unwired: 2 in, 2 out]
            n141 = property on="SAVE" class="Bool"("DisabledEnum"=w168) -> ()  [unwired: 2 in, 2 out]
            "Hardware Running?" <- TRUE ("Run Running?")
          }
          frame "Hardware Stop" {
            n142 = Flush Queue(queue=w183) -> (queue out=w182:refnum<queue>)  [unwired: 1 in, 2 out]
            n143 = Enqueue Element(queue=w182, element=T16 {"Action"=enum."Stop", "Data"=variant}) -> ()  [unwired: 2 in, 3 out]
            n144 = call "HardwareAbortGlobal.vi"("Action"=HardwareAbortGlobalAction."Set", "Set Value"=TRUE) -> ()  [unwired: 9 in, 1 out]
          }
          frame "Hardware Stopped" {
            w187 = T13."Enabled" ("Disabled")
            n145 = local write "Hardware Running?"(FALSE ("Hardware Armed?")) -> ()
            n146 = Enqueue Element(queue=w192, element=T14 {"Action"=enum."Log Stop", "Data"=variant}, error in (no error)=w191) -> (error out=w190:errorcluster)  [unwired: 1 in, 2 out]
            n147 = property on="LOG START" class="Bool (strict)"("DisabledEnum"=T13."Disabled and Grayed Out" ("Disabled")) -> ()  [unwired: 2 in, 2 out]
            n148 = property on="SHOW DUT DIALOG" class="Bool"("DisabledEnum"=w187) -> ()  [unwired: 2 in, 2 out]
            n149 = property on="SHOW LOG DIALOG" class="Bool"("DisabledEnum"=w187) -> ()  [unwired: 2 in, 2 out]
            n150 = property on="SHOW MEASURE DIALOG" class="Bool"("DisabledEnum"=w187) -> ()  [unwired: 2 in, 2 out]
            n151 = property on="SHOW SOURCE DIALOG" class="Bool"("DisabledEnum"=w187) -> ()  [unwired: 2 in, 2 out]
            n152 = property on="SHOW TRIGGER DIALOG" class="Bool"("DisabledEnum"=w187) -> ()  [unwired: 2 in, 2 out]
            n153 = property on="OPEN" class="Bool"("DisabledEnum"=w187) -> ()  [unwired: 2 in, 2 out]
            n154 = property on="RESET" class="Bool"("DisabledEnum"=w187) -> ()  [unwired: 2 in, 2 out]
            n155 = property on="SAVE" class="Bool"("DisabledEnum"=w187) -> ()  [unwired: 2 in, 2 out]
          }
          frame "Log Start" {
            n156 = Flush Queue(queue=w197) -> (queue out=w196:refnum<queue>)  [unwired: 1 in, 2 out]
            n157 = Enqueue Element(queue=w196, element=T19 {"Action"=enum."Create", "Data"=variant}) -> ()  [unwired: 2 in, 3 out]
          }
          frame "Log Arm" {
            n158 = Flush Queue(queue=w202) -> (queue out=w203:refnum<queue>)  [unwired: 1 in, 2 out]
            n159 = Enqueue Element(queue=w203, element=T19 {"Action"=enum."Start", "Data"=variant}) -> ()  [unwired: 2 in, 3 out]
          }
          frame "Log Started" {
            w208 = TRUE ("Log Running?")
            n160 = call "SetupGlobal.vi"("Action"=SetupGlobalAction."Get") -> ("Value Out"=w206:T23)  [unwired: 10 in]
            n161 = Variant To Data(type=path "", Variant=w212) -> (data=→"Log File":path)  [unwired: 1 in, 1 out]
            n162 = Unbundle By Name(w206) -> ("Log.Stop.Trigger Type"=w205:T33)
            n163 = case shown="\"Timer\"" w205 {
              tunnel: [T13."Disabled and Grayed Out" ("Disabled") T13."Enabled" ("Disabled") T13."Enabled" ("Disabled") T13."Enabled" ("Disabled") T13."Enabled" ("Disabled")] -> w209
              frame "None", Default {
              }
              frame "User" {
              }
              frame "Timer" {
              }
              frame "File Size" {
              }
              frame "Digital IO" {
              }
            }
            n164 = local write "LOG START"(w208) -> ()
            n165 = property on="LOG START" class="Bool (strict)"("DisabledEnum"=w209) -> ()  [unwired: 2 in, 2 out]
            "Log Running?" <- w208
          }
          frame "Log Stop" {
            n166 = Flush Queue(queue=w223) -> (queue out=w222:refnum<queue>, error out=w221:errorcluster)  [unwired: 1 in, 1 out]
            n167 = Enqueue Element(queue=w222, element=T19 {"Action"=enum."Stop", "Data"=variant}, error in (no error)=w221) -> ()  [unwired: 1 in, 3 out]
          }
          frame "Log Stopped" {
            w230 = FALSE ("Log Running?")
            n168 = call "SetupGlobal.vi"("Action"=SetupGlobalAction."Get") -> ("Value Out"=w228:T23)  [unwired: 10 in]
            n169 = Unbundle By Name(w228) -> ("Log.Start.Trigger Type"=w226:T28)
            n170 = case shown="\"User\"" w226 {
              tunnel: [T13."Disabled and Grayed Out" ("Disabled") w235 T13."Disabled and Grayed Out" ("Disabled") T13."Disabled and Grayed Out" ("Disabled")] -> w229
              frame "Immediate", Default {
              }
              frame "User" {
                n171 = local read "Hardware Running?"() -> (w238:bool)
                n172 = Select(t=T13."Enabled" ("Disabled"), s=w238, f=T13."Disabled and Grayed Out") -> (s? t:f=w235:T13)
              }
              frame "Timer" {
              }
              frame "Digital IO" {
              }
            }
            n173 = local write "Log Running?"(w230) -> ()
            n174 = local write "LOG START"(w230) -> ()
            n175 = local write "Log File"(path "") -> ()
            n176 = property on="LOG START" class="Bool (strict)"("DisabledEnum"=w229) -> ()  [unwired: 2 in, 2 out]
          }
          frame "Create Chart" {
            n177 = call "DisplayDataChartDialogGlobal.vi"("Action"=DisplayDataChartDialogGlobalAction."Create") -> ()  [unwired: 11 in]
          }
          frame "Error" {
            n178 = Variant To Data(type=w245, Variant=w246) -> (data=w244:errorcluster)  [unwired: 1 in, 1 out]
            n179 = call <vilib>:"General Error Handler.vi"("error in (no error)"=w244) -> ()  [unwired: 10 in, 5 out]
          }
          frame "Shutdown" {
            n180 = Release Queue(queue=w260, error in (no error)=w259) -> (error out=w258:errorcluster)  [unwired: 1 in, 2 out]
            n181 = Flush Queue(queue=w257) -> (queue out=w252:refnum<queue>)  [unwired: 1 in, 2 out]
            n182 = Flush Queue(queue=w255) -> (queue out=w254:refnum<queue>)  [unwired: 1 in, 2 out]
            n183 = Not(x=w262) -> (.not. x?=w261:bool)
            n184 = local read "Hardware START"() -> (w251:bool)
            n185 = Enqueue Element(queue=w254, element=T19 {"Action"=enum."Shutdown", "Data"=variant}) -> ()  [unwired: 2 in, 3 out]
            n186 = case shown="True" w251 {
              tunnel: w252 -> [w263 w265]
              tunnel: [w263 w264] -> w250
              frame False {
              }
              frame True {
                n187 = Enqueue Element(queue=w265, element=T16 {"Action"=enum."Stop", "Data"=variant}) -> (queue out=w264:refnum<queue>)  [unwired: 2 in, 2 out]
              }
            }
            n188 = call "DisplayDataChartDialogGlobal.vi"("Action"=DisplayDataChartDialogGlobalAction."Close All") -> ()  [unwired: 11 in]
            n189 = call "SetupGlobal.vi"("Action"=SetupGlobalAction."Reset") -> ()  [unwired: 10 in, 1 out]
            n190 = Enqueue Element(queue=w250, element=T16 {"Action"=enum."Shutdown", "Data"=variant}) -> ()  [unwired: 2 in, 3 out]
          }
        }
      }
      n191 = Merge Errors(w27, w24) -> (w26:errorcluster)
    }
    frame Error {
    }
  }
  n192 = call "HardwareLoop.vi"("Error In"=w8, "Executable Configuration"=w3, "Data Structures"=w6, "Action Queues"=w7) -> ("Error Out"=w11:errorcluster)  [unwired: 7 in]
  n193 = call "LogLoop.vi"("Error In"=w8, "Executable Configuration"=w3, "Data Structures"=w6, "Action Queues"=w7) -> ("Error Out"=w5:errorcluster)  [unwired: 7 in]
  n194 = Merge Errors(w13, w11, w5) -> (w12:errorcluster)
  n195 = call "Shutdown.vi"("Error In"=w12) -> ()  [unwired: 10 in, 1 out]
